vi "Move Relative.vi"(7 "Axes":string, 8 "Error In":errorcluster, 9 "Units":string, 11 "GPIB address in":string) -> (0 "Error Out":errorcluster, 3 "GPIB address out":string)   [LabVIEW 2014]
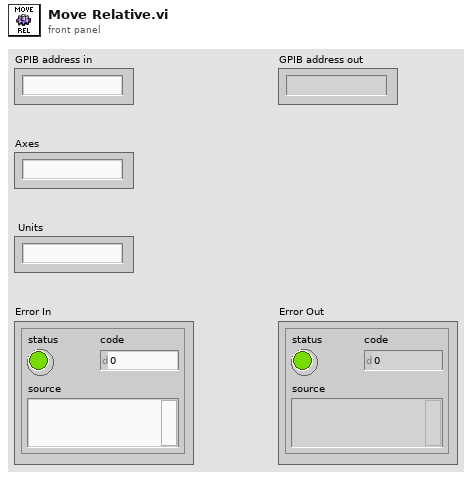
[diagram p1: front panel]
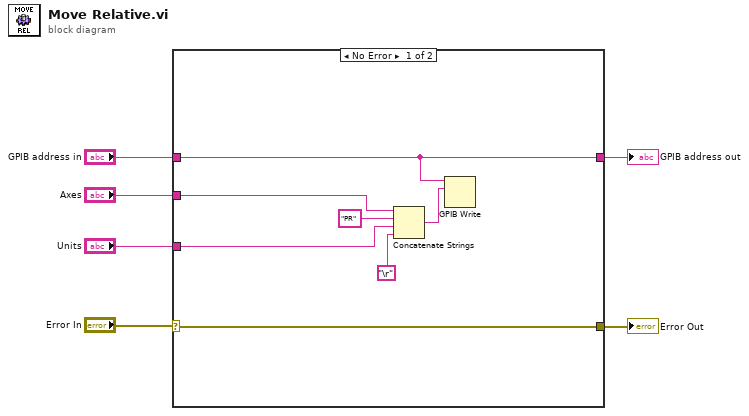
[diagram p0: block diagram]
diagram:
  n1 = case shown="No Error" "Error In" {
    selector: "Error In" -> [w10 w15]
    tunnel: [w10 w15] -> w5
    tunnel: "GPIB address in" -> [w7 w14]
    tunnel: [w7 w14] -> w3
    tunnel: "Axes" -> [w8 _]
    tunnel: "Units" -> [w9 _]
    frame No Error {
      n2 = Concatenate Strings(w8, "PR" ("data"), w9, "\r") -> (w11:string)
      n3 = GPIB Write(0:w7, 1:w11) -> ()  [unwired: 3 in, 2 out]
    }
    frame Error {
    }
  }
  "Error Out" <- w5
  "GPIB address out" <- w3
